vi "Get Shared Variable Channel Info.vi"(8 "error in (no error)":errorcluster, 9 "IP Address":string, 10 "Section GUID":string, 11 "Device Ref in":T3 format="%.0x") -> (0 "error out":errorcluster, 2 "Shared Variable Channel Info":T1, 3 "Device Ref out":T3 format="%.0x")   [LabVIEW 2012, in "Shared Variable Custom Device.lvlib"]
uses:
  Shared Variable Custom Device.lvlib
  <vilib>/NI Veristand/Custom Device API/Custom Device Item Ref.ctl
  RTMs/Existing Channel Data.ctl
  <vilib>/Utility/VariantDataType/Type.ctl
  <vilib>/NI Veristand/Custom Device Tools/Custom Device Utility Library/NI VeriStand - Search for Item by GUID.vi
  <vilib>/NI Veristand/Custom Device Tools/Custom Device Utility Library/Custom Device Utility Library.lvlib
  <vilib>/Utility/VariantDataType/VariantType.lvlib
  <vilib>/NI Veristand/Custom Device API/Custom Device API.lvlib
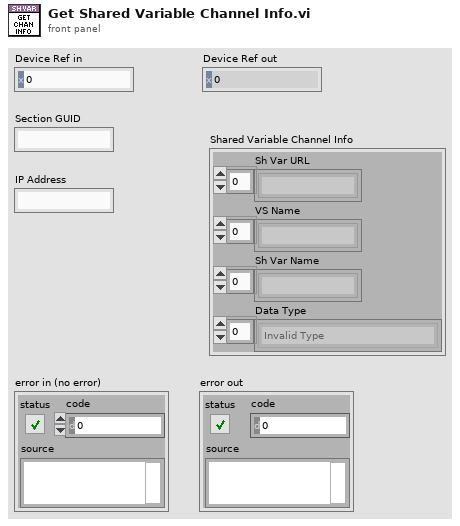
[diagram p1: front panel]
types:
  T1 = typedef "Shared Variable Custom Device.lvlib/Existing Channel Data.ctl" = cluster{"Sh Var URL":string[], "VS Name":string[], "Sh Var Name":string[], "Data Type":T2[]}
  T2 = typedef "VariantType.lvlib/Type.ctl" = enum8{"Invalid Type", "Void", "I8", "I16", "I32", "I64", "U8", "U16", "U32", "U64", "Single Float", "Double Float", "Extended Float", "Single Complex", "Double Complex", "Extended Complex", "Enum U8", "Enum U16", "Enum U32", "Enum U64", "Single Float With Unit", "Double Float With Unit", "Extended Float With Unit", "Single Complex with Unit", "Double Complex with Unit", "Extended Complex with Unit", "Boolean", "String", "Path", "Picture", "Tag", "Array", "Cluster", "Variant", "LV Variant", "Waveform", "Timestamp", "Digital Waveform", "Digital Data", "ExpressData", "Refnum", "External Data", "VI", "Poly VI", "LabVIEW Class Instance", "Fixed Point"}
  T3 = typedef "Custom Device API.lvlib/Custom Device Item Ref.ctl" = u64
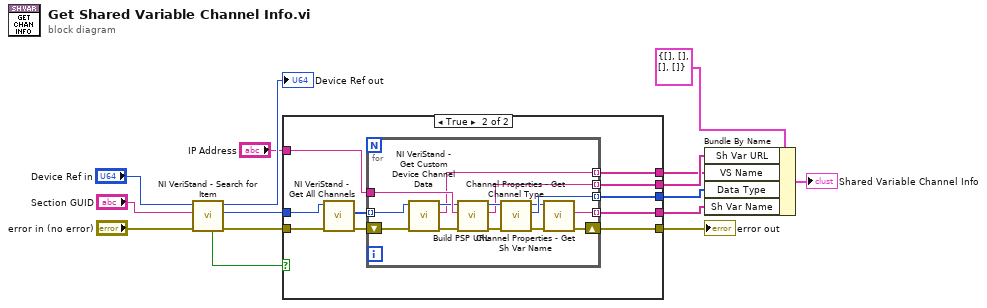
[diagram p0: block diagram]
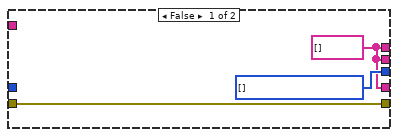
[diagram p2: hidden frame]
diagram:
  n1 = call-poly <vilib>:"NI VeriStand - Search for Item.vi"("error in"="error in (no error)", "Item GUID"="Section GUID", "Section Ref in"="Device Ref in") -> ("error out"=w10:errorcluster, "Item Ref"=w11:T3, "Section Ref out"=→"Device Ref out":T3, "Found"=w9:bool)  [unwired: 5 in]
  n2 = case shown="True" w9 {
    tunnel: w10 -> [w18 w27]
    tunnel: w11 -> [_ w28]
    tunnel: [w18 w24] -> w12
    tunnel: "IP Address" -> [_ w23]
    tunnel: [w17 w22] -> w4
    tunnel: [w16 w21] -> w6
    tunnel: [w16 w20] -> w3
    tunnel: [w16 w19] -> w2
    frame False {
      w17 = T2[] [] items=["Invalid Type", "Void", "I8", "I16", "I32", "I64", "U8", "U16", "U32", "U64", "Single Float", "Double Float", "Extended Float", "Single Complex", "Double Complex", "Extended Complex", "Enum U8", "Enum U16", "Enum U32", "Enum U64", "Single Float With Unit", "Double Float With Unit", "Extended Float With Unit", "Single Complex with Unit", "Double Complex with Unit", "Extended Complex with Unit", "Boolean", "String", "Path", "Picture", "Tag", "Array", "Cluster", "Variant", "LV Variant", "Waveform", "Timestamp", "Digital Waveform", "Digital Data", "ExpressData", "Refnum", "External Data", "VI", "Poly VI", "LabVIEW Class Instance", "Fixed Point"]
      w16 = string[] []
    }
    frame True {
      n3 = call <vilib>:"NI VeriStand - Get All Channels.vi"("error in"=w27, "Section Ref in"=w28) -> ("error out"=w25:errorcluster, "Channel Refs"=w26:T3[])  [unwired: 6 in, 2 out]
      n4 = for {
        tunnel: w26 -> [w36] mode=indexing
        shift-right: [w30] -> w24
        shift-left: w25 -> [w37]
        tunnel: w23 -> [w42]
        tunnel: [w33] -> w20 mode=indexing
        tunnel: [w38] -> w22 mode=indexing
        tunnel: [w39] -> w21 mode=indexing
        tunnel: [w29] -> w19 mode=indexing
        n5 = call <vilib>:"NI VeriStand - Get Custom Device Channel Data.vi"("error in (no error)"=w37, "Channel Ref in"=w36) -> ("error out"=w34:errorcluster, "Channel Name"=w33:string, "Channel Ref out"=w35:T3)  [unwired: 4 in, 3 out]
        n6 = call "Build PSP URL.vi"("error in (no error)"=w34, "IP Address"=w42, "Channel Ref in"=w35) -> ("error out"=w40:errorcluster, "Shared Variable URL"=w39:string, "Channel Ref out"=w41:T3)  [unwired: 6 in]
        n7 = call "Channel Properties - Get Channel Type.vi"("error in (no error)"=w40, "Channel Ref in"=w41) -> ("error out"=w31:errorcluster, "Channel Type"=w38:T2, "Channel Ref out"=w32:T3)  [unwired: 7 in]
        n8 = call "Channel Properties - Get Sh Var Name.vi"("error in (no error)"=w31, "Channel Ref in"=w32) -> ("error out"=w30:errorcluster, "Shared Variable Name"=w29:string)  [unwired: 7 in, 1 out]
      }
    }
  }
  "error out" <- w12
  n9 = Bundle By Name(cluster=T1 {"Sh Var URL"=[], "VS Name"=[], "Sh Var Name"=[], "Data Type"=[]} ("Shared Variable Channel Info"), "Sh Var URL"=w6, "VS Name"=w3, "Data Type"=w4, "Sh Var Name"=w2) -> (→"Shared Variable Channel Info":T1)
